vi "Do.vi"(8 "error in":errorcluster, 10 "Actor in":refnum<class "Actor.lvclass">, 11 "Change Denuder State MSG":refnum<class "Change Denuder State MSG.lvclass">) -> (0 "error out":errorcluster, 2 "Actor out":refnum<class "Actor.lvclass">)   [LabVIEW 2014, in "Controller.lvlib" / "Change Denuder State MSG.lvclass"]
doc: "(<B>Filename</B>: Actor Framework.lvlib:Message.lvclass:Do.vi)\n\nDefines what a message does when it is received by an actor. Generally, a message instructs an actor to invoke one of its methods. By default, this method does nothing. A child class must override it to define behavior. Create a child class by using the Actor Framework Message Maker dialog box."
uses:
  Change Denuder State MSG.lvclass
  <vilib>/ActorFramework/Actor/Actor.lvclass
  Change Denuder State MSG.lvclass/Change Denuder State MSG.ctl
  Controller.lvclass
  SuperActor/SuperClass.lvclass/SuperClass.ctl
  SuperActor/Read Log Session.vi
  SuperActor/Read CVT Session.vi
  <vilib>/DAQmx/write.llb/DAQmx Write (Digital Bool 1Line 1Point).vi
  <vilib>/DAQmx/write.llb/DAQmx Write (Digital 1D Bool NChan 1Samp 1Line).vi
  <userlib>/_Session Fwk/Session - Root.lvclass
  reusable/Session APIs/Session Log/System Log.lvclass
  reusable/Session APIs/CVT/CVT.lvclass
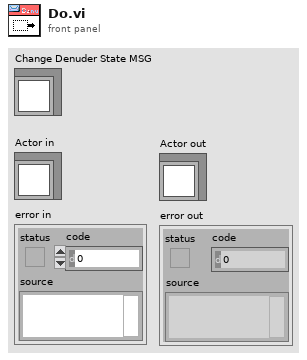
[diagram p1: front panel]
types:
  T1 = typedef "Session - Root.lvclass/Session Handle.ctl" = refnum<data-value>
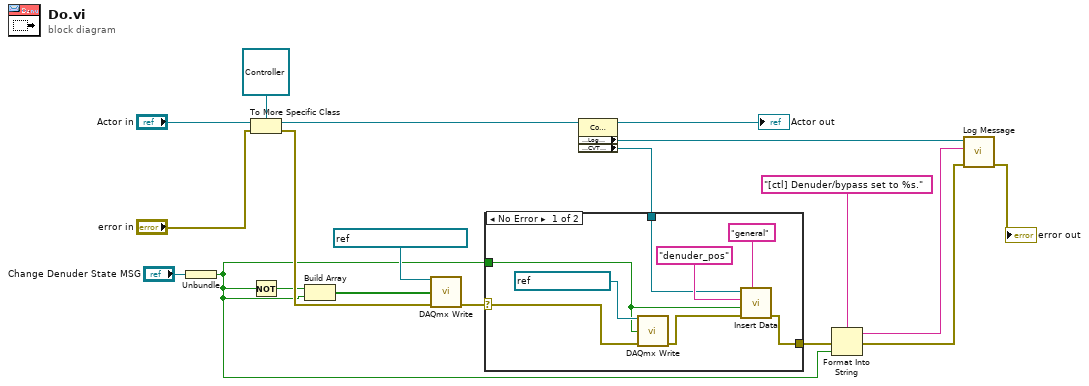
[diagram p0: block diagram]
diagram:
  n1 = Unbundle("Change Denuder State MSG") -> (w2:bool)
  n2 = To More Specific Class(target class=refnum<class "Controller.lvclass"> refnum ("Controller:Controller"), reference="Actor in", error in="error in") -> (specific class reference=w13:refnum<class "Controller.lvclass">, error out=w11:errorcluster)
  n3 = Not(x=w2) -> (.not. x?=w1:bool)
  n4 = Build Array(w1, w2) -> (w16:bool[])
  n5 = call-poly <vilib>:"DAQmx Write.vi"("task/channels in"=refnum<k21> "Denuder Valve CMD", "data"=w16, "error in"=w11) -> ("error out"=w19:errorcluster)  [unwired: 10 in, 2 out]
  n6 = property class="Controller"(reference=w13) -> (reference out=→"Actor out":refnum<class "Controller.lvclass">, "Accessors:Log Session"=w9:T1, "Accessors:CVT Session"=w3:T1)  [unwired: 1 in, 1 out]
  n7 = case shown="No Error" w19 {
    selector: w19 -> [w26 w28]
    tunnel: [w20 w28] -> w4
    tunnel: w2 -> [w22 _]
    tunnel: w3 -> [w23 _]
    frame No Error {
      n8 = call-poly <vilib>:"DAQmx Write.vi"("task/channels in"=refnum<k21> "Denuder LED", "data"=w22, "error in"=w26) -> ("error out"=w21:errorcluster)  [unwired: 10 in, 2 out]
      n9 = call "Insert Data.vi"("Group"="general", "error in"=w21, "Data"=w22, "tag"="denuder_pos", "CVT Session In"=w23) -> ("error out"=w20:errorcluster)  [unwired: 5 in, 1 out]
    }
    frame Error {
    }
  }
  n10 = Format Into String(format string="[ctl] Denuder/bypass set to %s.", error in=w4, w2) -> (resulting string=w7:string, error out=w6:errorcluster)  [unwired: 1 in]
  n11 = call "Log Message.vi"("error in"=w6, "MSG In"=w7, "session in"=w9) -> ("error out"=→"error out":errorcluster)  [unwired: 7 in, 1 out]
